vi "SortZtoA.vi"(0 "Input Array":string[](array[string]), 11 "error in":errorcluster) -> (4 "reversed array":string[](array[string]), 15 "error out":errorcluster)   [LabVIEW 2023, in "Unit Testing CA1.lvlib"]
uses:
  Unit Testing CA1.lvlib
  46095cf5-40be-4930-a84a-d385456607c1.vi
  <vilib>/Comparison/Less/Less Functor/Less Functor.lvclass
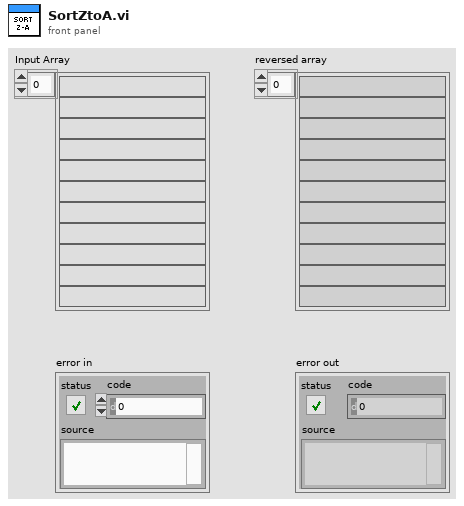
[diagram p1: front panel]
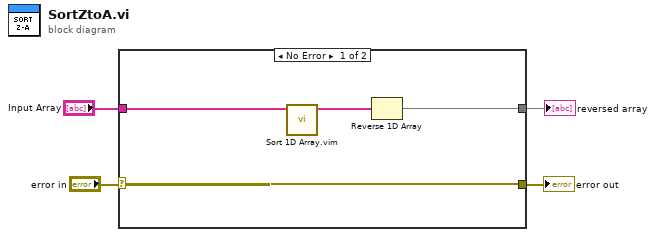
[diagram p0: block diagram]
diagram:
  n1 = case shown="No Error" "error in" {
    selector: "error in" -> [w8 w10]
    tunnel: [w8 w10] -> w3
    tunnel: "Input Array" -> [w6 w9]
    tunnel: [w5 w9] -> w1
    frame No Error {
      n2 = call "Sort 1D Array.vim"("unsorted array"=w6) -> ("sorted array"=w7:string[])  [unwired: 10 in]
      n3 = Reverse 1D Array(array=w7) -> (reversed array=w5:string[])
    }
    frame Error {
    }
  }
  "error out" <- w3
  "reversed array" <- w1
